vi "Generate Assert VI Template Path.vi"(7 "Data Type":T1, 8 "error in (no error)":errorcluster, 9 "Operation":string) -> (0 "error out":errorcluster, 2 "Template Path":path)   [LabVIEW 2016]
uses:
  <vilib>/Utility/Data Type/Type Definitions/Data Type.ctl
  <vilib>/Utility/Data Type/NI_Data Type.lvlib
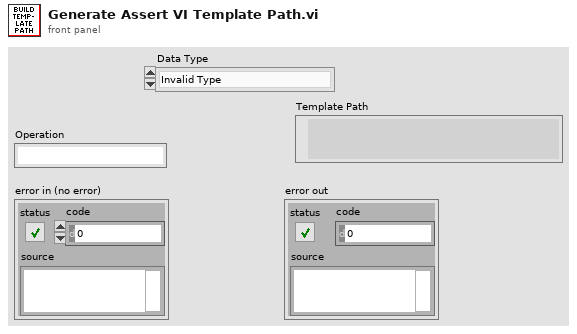
[diagram p1: front panel]
types:
  T1 = typedef "NI_Data Type.lvlib/Data Type.ctl" = enum8{"Invalid Type", "Void", "I8", "I16", "I32", "I64", "U8", "U16", "U32", "U64", "Single Float", "Double Float", "Extended Float", "Single Complex", "Double Complex", "Extended Complex", "Enum U8", "Enum U16", "Enum U32", "Enum U64", "Single Float With Unit", "Double Float With Unit", "Extended Float With Unit", "Single Complex with Unit", "Double Complex with Unit", "Extended Complex with Unit", "Boolean", "String", "Path", "Picture", "Tag", "Array", "Cluster", "Variant", "LV Variant", "Waveform", "Timestamp", "Digital Waveform", "Digital Data", "ExpressData", "Refnum", "External Data", "VI", "Poly VI", "LabVIEW Class Instance", "Fixed Point"}
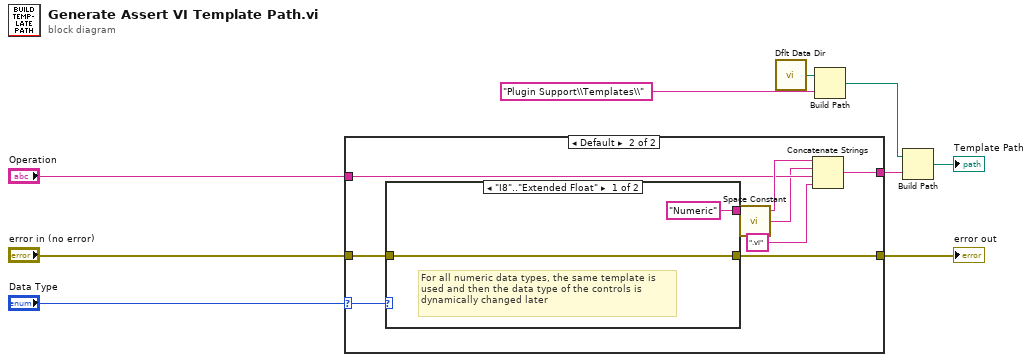
[diagram p0: block diagram]
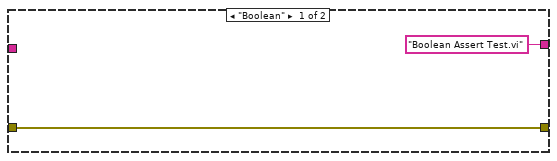
[diagram p2: hidden frame]
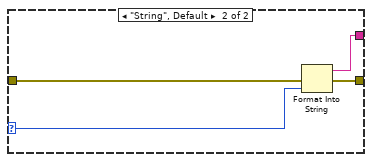
[diagram p3: hidden frame]
diagram:
  n1 = case shown="Default" "Data Type" {
    selector: "Data Type" -> [_ w17]
    tunnel: [w10 w19] -> w9
    tunnel: "error in (no error)" -> [w10 w18]
    tunnel: "Operation" -> [_ w14]
    tunnel: ["Boolean Assert Test.vi" w12] -> w3
    frame "Boolean" {
    }
    frame Default {
      n2 = case shown="\"I8\"..\"Extended Float\"" w17 {
        selector: w17 -> [_ w23]
        tunnel: [w20 w25] -> w19
        tunnel: w18 -> [w20 w24]
        tunnel: ["Numeric" w22] -> w16
        frame "I8".."Extended Float" {
          # "For all numeric data types, the same template is used and then the data type of the controls is dynamically changed later"
        }
        frame "String", Default {
          n3 = Format Into String(error in=w24, w23) -> (resulting string=w22:string, error out=w25:errorcluster)  [unwired: 2 in]
        }
      }
      n4 = call <vilib>:"Space Constant.vi"() -> ("String"=w13:string)
      n5 = Concatenate Strings(w16, w13, w14, ".vi") -> (w12:string)
    }
  }
  "error out" <- w9
  n6 = call <vilib>:"Dflt Data Dir.vi"() -> ("App:Default Data Directory"=w2:path)
  n7 = Build Path(base path=w2, name or relative path="Plugin Support\\Templates\\") -> (appended path=w5:path)
  n8 = Build Path(base path=w5, name or relative path=w3) -> (appended path=→"Template Path":path)
